vi "Read-all-variables.vi"(8 "error in (no error)":errorcluster, 11 "Correct. params. ref. in":refnum<data-value>) -> (0 "error out":errorcluster, 2 "Correct. vars.":T1, 3 "Correct. params. ref.":refnum<data-value>)   [LabVIEW 2013, in "CameraVision.lvlib" / "CV-Correction.lvclass"]
uses:
  CV-Correction.lvclass
  Correction-variables.ctl
  CV-Correction.lvclass/CV-Correction.ctl
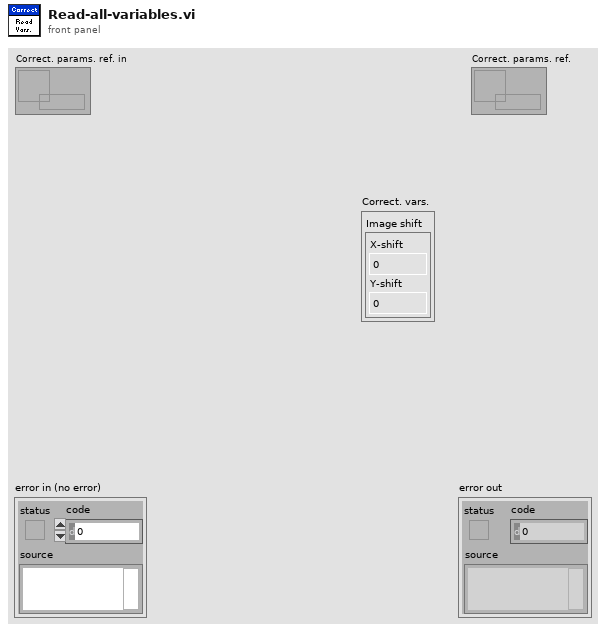
[diagram p1: front panel]
types:
  T1 = typedef "CameraVision.lvlib/CV-Correction.lvclass/Correction-variables.ctl" = cluster{"Image shift":cluster{"X-shift":i32, "Y-shift":i32}}
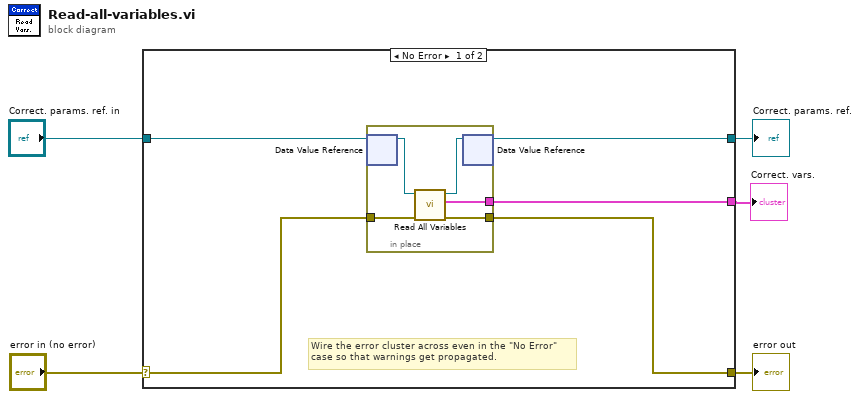
[diagram p0: block diagram]
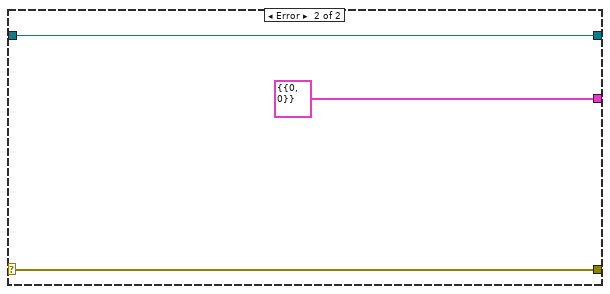
[diagram p2: hidden frame]
diagram:
  n1 = case shown="No Error" "error in (no error)" {
    selector: "error in (no error)" -> [w8 w18]
    tunnel: [w10 w18] -> w4
    tunnel: "Correct. params. ref. in" -> [w7 w16]
    tunnel: [w9 T1 {"Image shift"={"X-shift"=0, "Y-shift"=0}} ("Correct. vars.")] -> w2
    tunnel: [w6 w16] -> w1
    frame No Error {
      # "Wire the error cluster across even in the \"No Error\"\ncase so that warnings get propagated."
      n2 = in-place {
        in-place-border: [w15] -> w10
        in-place-border: [w14] -> w9
        in-place-border: w8 -> [w13]
        n3 = in-place-dvr #1(w7) -> (w11:refnum<class "CV-Correction.lvclass">)  [unwired: 1 out]
        n4 = call "Read All Variables.vi"("error in (no error)"=w13, "Correct params in"=w11) -> ("error out"=w15:errorcluster, "Correct. vars."=w14:T1, "Correct params out"=w12:refnum<class "CV-Correction.lvclass">)  [unwired: 7 in]
        n5 = in-place-dvr #1(w12) -> (w6:refnum<data-value>)  [unwired: 1 out]
      }
    }
    frame Error {
    }
  }
  "error out" <- w4
  "Correct. params. ref." <- w1
  "Correct. vars." <- w2
